vi "RD Digital I2C Tx Rx IO Set.vi"(8 "error in (no error)":errorcluster caption="错误输入（无错误）", 9 "SDADIO":i32, 10 "SCLDIO":i32, 11 "handle":u64) -> (0 "error out":errorcluster caption="错误输出", 2 "function return":i32, 3 "handle out":u64)   [LabVIEW 2018, in "InstrumentsPlayground.lvlib"]
doc: "CLIFFAPI int CliffDigitalI2CRateSet(FT_HANDLE handle, double rate); CLIFFAPI int CliffDigitalI2CTxRxIOSet(FT_HANDLE handle, int SCLDIO, int SDADIO);"
uses:
  InstrumentsPlayground.lvlib
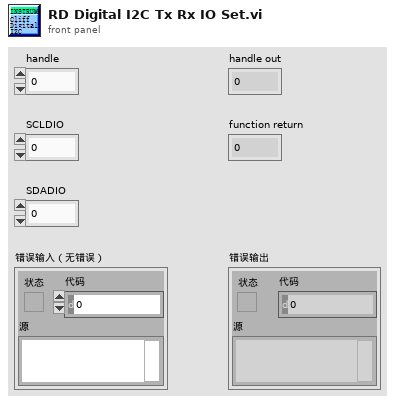
[diagram p1: front panel]
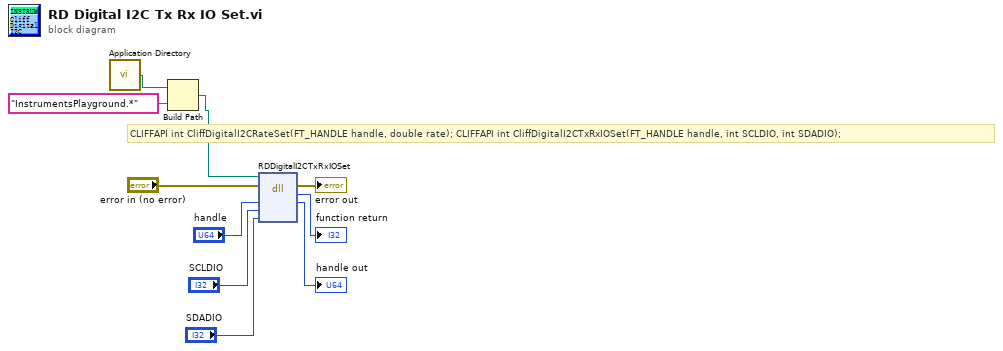
[diagram p0: block diagram]
diagram:
  # "CLIFFAPI int CliffDigitalI2CRateSet(FT_HANDLE handle, double rate); CLIFFAPI int CliffDigitalI2CTxRxIOSet(FT_HANDLE handle, int SCLDIO, int SDADIO);"
  n1 = call <vilib>:"Application Directory.vi"() -> ("Application Directory"=w2:path)
  n2 = Build Path(base path=w2, name or relative path="InstrumentsPlayground.*" ("名称或相对路径")) -> (appended path=w1:path)
  n3 = dll-call lib="E:/Work/YZCourse_Xtext/Cliff/API/IPLabView lib/InstrumentsPlayground.*" fn="RDDigitalI2CTxRxIOSet"(path in=w1, error in="error in (no error)", "handle"="handle", "SCLDIO"="SCLDIO", "SDADIO"="SDADIO") -> (error out=→"error out":errorcluster, "返回类型"=→"function return":i32, "handle"=→"handle out":u64)  [unwired: 3 in, 1 out]
